vi "Check if Data Type has User-Definable String.vi"(1 "EasyXML Type":T1=enum."Cluster") -> (0 "Has User-Definable String Data?":bool)   [LabVIEW 2011]
uses:
  Type Defs/Formatting Data Type -- Enum.ctl
panel:
  # "OpenG Format Generic Data to XML Value.vi  - formats the data of scalar data\n\nCopyright (C) 2004, 2003 Jim Kring jim@jimkring.com\n\nThis library is free software; you can redistribute it and/or\nmodify it under the terms of the GNU Lesser General Public\nLicense as published by the Free Software Foundation; either\nversion 2.1 of the License, or (at your option) any later version.\nThis library is distributed in the hope that it will be useful,\nbut WITHOUT ANY WARRANTY; without even the implied warranty of\nMERCHANTABILITY or FITNESS FOR A PARTICULAR PURPOSE. See the GNU\nLesser General Public License for more details.\nYou should have received a copy of the GNU Lesser General Public\nLicense along with this library; if not, write to the Free Software\nFoundation, Inc., 59 Temple Place, Suite 330, Boston, MA 02111-1307 USA"
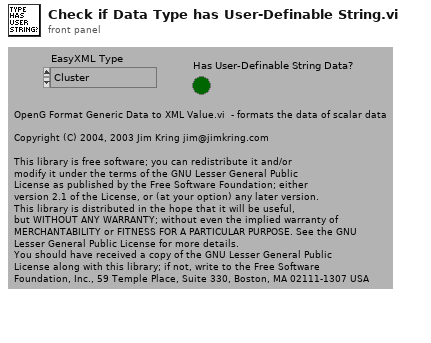
[diagram p1: front panel]
types:
  T1 = typedef "Formatting Data Type -- Enum.ctl" = enum16{"<unknown>", "Cluster", "Array", "String", "Path", "Boolean", "Time Stamp", "Enum", "Numeric - EXT", "Numeric - DBL", "Numeric - SGL", "Numeric - I64", "Numeric - I32", "Numeric - I16", "Numeric - I8", "Numeric - U64", "Numeric - U32", "Numeric - U16", "Numeric - U8", "Numeric - CXT", "Numeric - CDB", "Numeric - CSG", "VISA Resource"}
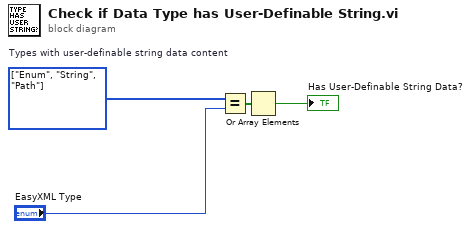
[diagram p0: block diagram]
diagram:
  w1 = T1[] [enum."Enum", enum."String", enum."Path"] items=["<unknown>", "Cluster", "Array", "String", "Path", "Boolean", "Time Stamp", "Enum", "Numeric - EXT", "Numeric - DBL", "Numeric - SGL", "Numeric - I64", "Numeric - I32", "Numeric - I16", "Numeric - I8", "Numeric - U64", "Numeric - U32", "Numeric - U16", "Numeric - U8", "Numeric - CXT", "Numeric - CDB", "Numeric - CSG", "VISA Resource"]  # Types with user-definable string data content
  n1 = Equal?(x=w1, y="EasyXML Type") -> (x = y?=w2:bool[])
  n2 = Or Array Elements(Boolean array=w2) -> (logical OR=→"Has User-Definable String Data?":bool)
